vi "探测器列表-修改网址.vi"(5 "元素名[]-探测器信息":string[](array[string]), 7 "table名-探测器列表":string, 8 "error in (no error)":errorcluster, 10 "修改网址":T1, 11 "数据库引用":T5) -> (0 "error out":errorcluster, 3 "数据库连接引用out":T5)   [LabVIEW 2017]
uses:
  <vilib>/addons/database/Connection.llb/Conn ObjectReference.ctl
  <vilib>/addons/database/NI_Database_API.lvlib
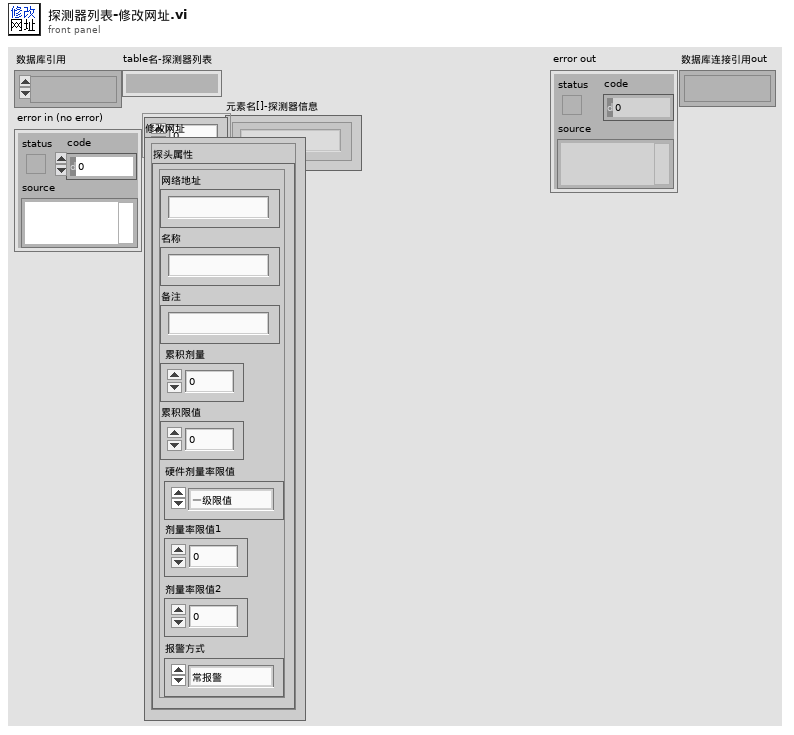
[diagram p1: front panel]
types:
  T1 = typedef "修改网址.ctl" = cluster{"探头属性":T2, "新网址":string}
  T2 = typedef "探测器信息.ctl" = cluster{"网络地址":string, "名称":string, "备注":string, "累积剂量":dbl, "累积限值":dbl, "硬件剂量率限值":T3, "剂量率限值1":dbl, "剂量率限值2":dbl, "报警方式":T4}
  T3 = typedef "探头剂量率限值选择.ctl" = enum16{"一级限值", "二级限值"}
  T4 = typedef "报警方式选择.ctl" = enum16{"常报警", "自动静音", "手动静音"}
  T5 = typedef "NI_Database_API.lvlib/Conn ObjectReference.ctl" = refnum<k1>
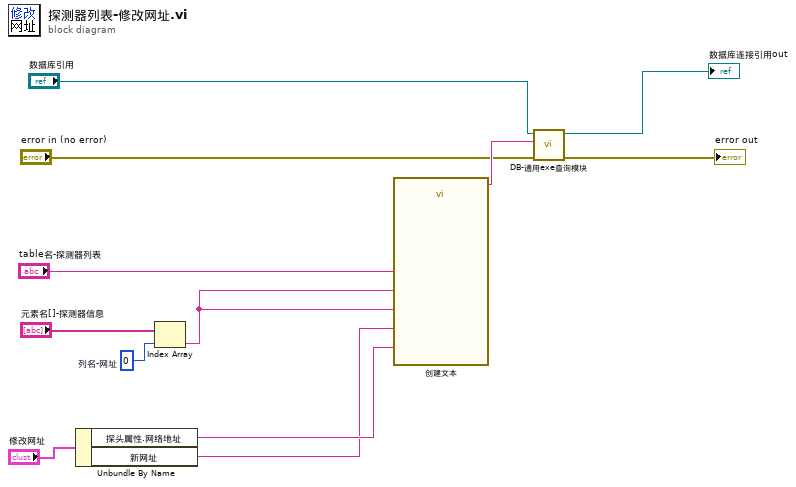
[diagram p0: block diagram]
diagram:
  w5 = 0  # 列名-网址
  n1 = Unbundle By Name("修改网址") -> ("探头属性.网络地址"=w2:string, "新网址"=w1:string)
  n2 = Index Array(array="元素名[]-探测器信息", index=w5) -> (element=w4:string)
  n3 = call "创建文本"("列名-网址1"=w4, "表名-设备表"="table名-探测器列表", "列名-网址"=w4, "新网址"=w1, "原网址"=w2) -> ("Result"=w12:string)  [unwired: 9 in, 1 out]
  n4 = call "DB-通用exe查询模块.vi"("error in (no error)"="error in (no error)", "SQL query"=w12, "数据库连接引用"="数据库引用") -> ("error out"=→"error out":errorcluster, "数据库连接引用out"=→"数据库连接引用out":T5)  [unwired: 4 in, 3 out]
